vi "Get Limits.vi"(8 "error in (no error)":errorcluster, 11 "Divider in":refnum<class "Divider.lvclass">) -> (0 "error out":errorcluster, 1 "Minimal sizes":i16[](array[numeric]), 2 "Maximal size":i16[](array[numeric]), 3 "Divider out":refnum<class "Divider.lvclass">)   [LabVIEW 2013, in "Divider.lvclass"]
doc: "Copyright 2018, Wiebe Walstra, wiebe@carya.nl."
uses:
  Divider.lvclass
  Divider.lvclass/Divider.ctl
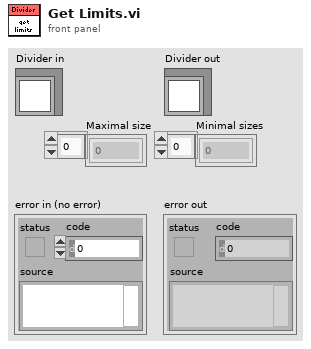
[diagram p1: front panel]
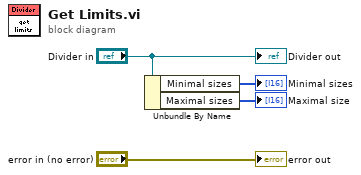
[diagram p0: block diagram]
diagram:
  n1 = Unbundle By Name("Divider in") -> ("Minimal sizes"=→"Minimal sizes":i16[], "Maximal sizes"=→"Maximal size":i16[])
  "error out" <- "error in (no error)"
  "Divider out" <- "Divider in"
